vi "ParStartTo.vi"(0 "ref in":u64, 1 "LocalTSAP":u16, 2 "Local Address":string="0.0.0.0", 11 "error in (no error)":errorcluster, 12 "Remote Address":string, 13 "RemoteTSAP":u16) -> (4 "ref out":u64, 6 "Result":i32, 15 "error out":errorcluster)   [LabVIEW 2010, in "Snap7.lvlib"]
uses:
  Snap7.lvlib
  windows/lv_snap7.dll
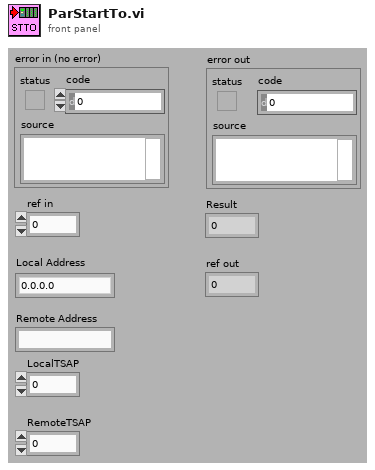
[diagram p1: front panel]
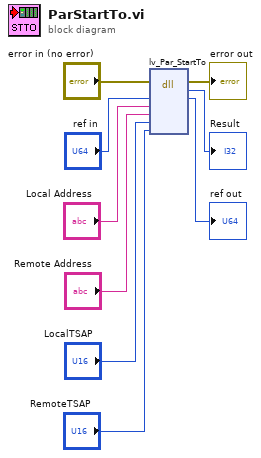
[diagram p0: block diagram]
diagram:
  n1 = dll-call lib="C:/snap7-src-1.0.0/LabVIEW/lib/windows/lv_snap7.dll" fn="lv_Par_StartTo"(error in="error in (no error)", "Partner"="ref in", "LocalAddress"="Local Address", "RemoteAddress"="Remote Address", "LocalTSAP"="LocalTSAP", "RemoteTSAP"="RemoteTSAP") -> (error out=→"error out":errorcluster, "return type"=→"Result":i32, "Partner"=→"ref out":u64)  [unwired: 6 in, 1 out]
